vi "writeSigleTime.vi"(8 "error in (no error)":errorcluster, 11 "试验时间":dbl) -> (0 "error out":errorcluster)   [LabVIEW 2014]
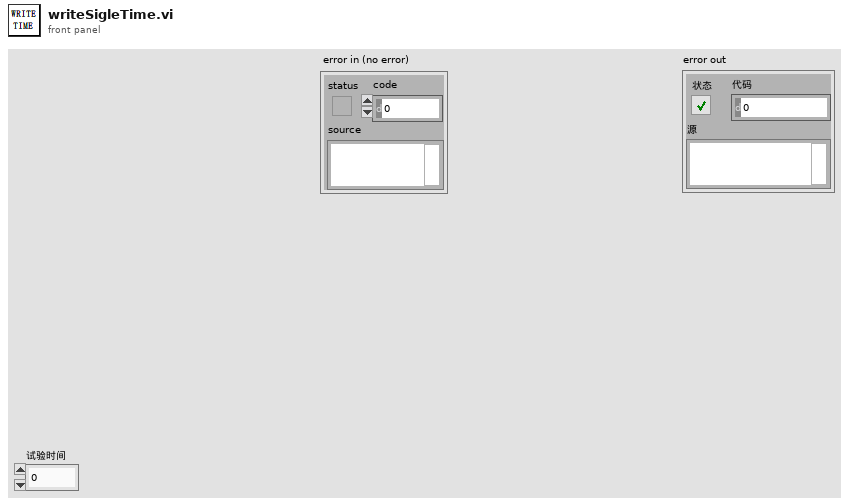
[diagram p1: front panel]
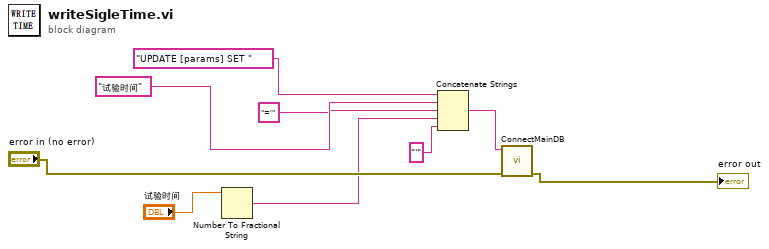
[diagram p0: block diagram]
diagram:
  n1 = Number To Fractional String(number="试验时间") -> (F-format string=w2:string)  [unwired: 3 in]
  n2 = Concatenate Strings("UPDATE [params] SET ", "试验时间" ("多行字符串"), "='", w2, "'") -> (w8:string)
  n3 = call "ConnectMainDB.vi"("error in (no error)"="error in (no error)", "SQL query"=w8) -> ("error out"=→"error out":errorcluster)  [unwired: 8 in, 1 out]
